vi "MSScript_Format_Start.vi"(9 "ValueArray":string[](array[string]), 10 "TagArray":string[](array[string]), 11 "MSScript in":refnum<class "MSScript.lvclass">) -> (0 "ValueErrorArray":bool[](array[boolean]), 1 "TagErrorArray":bool[](array[boolean]), 2 "ParamErrorArray":bool[](array[boolean]), 3 "Data":variant, 4 "#ofParamError":bool)   [LabVIEW 2018, in "MSScript.lvclass"]
uses:
  MSScript.lvclass
  Ctl/MSEditorParam RFStart.ctl
  MSScript.lvclass/MSScript.ctl
  MSScript_Transform_Extended.vi
  MSScript_Transform_UInt.vi
panel:
  in  "ParamValueType":T1={"freq"=0.001, "amp"=0.01, "wfmType"=0} {"amp" format="%#.3f"; "freq" format="%#.2f"}
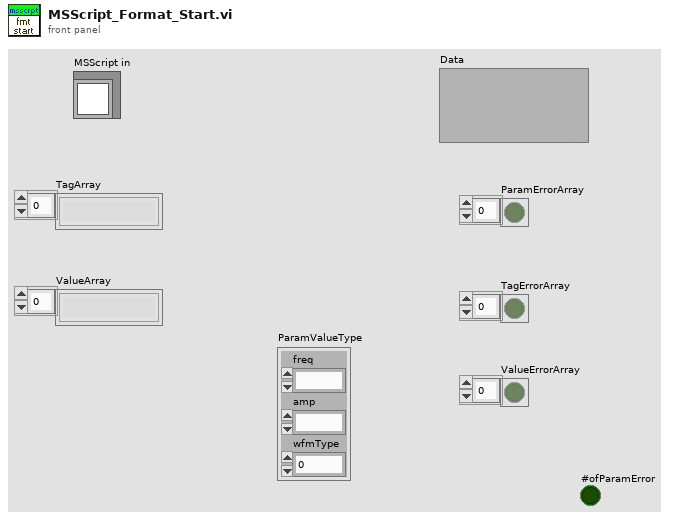
[diagram p1: front panel]
types:
  T1 = typedef "MSEditorParam RFStart.ctl" = cluster{"freq":ext, "amp":ext, "wfmType":u32}
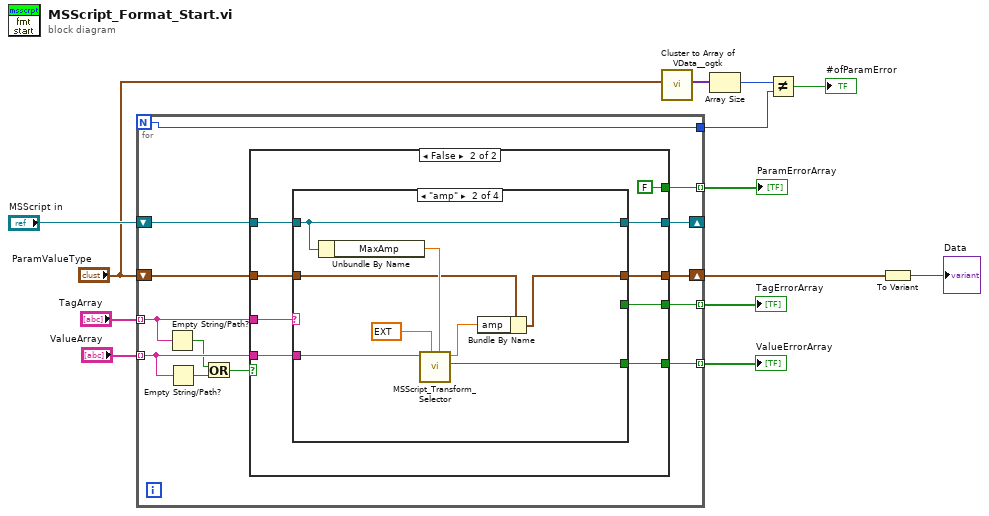
[diagram p0: block diagram]
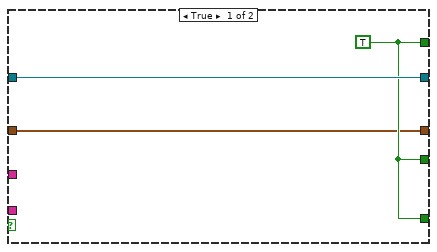
[diagram p2: hidden frame]
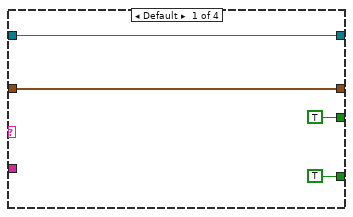
[diagram p3: hidden frame]
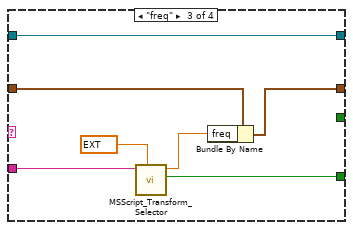
[diagram p4: hidden frame]
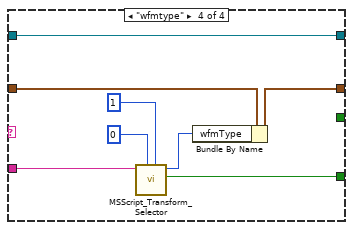
[diagram p5: hidden frame]
diagram:
  n1 = for {
    N -> [w14]
    tunnel: "TagArray" -> [w22] mode=indexing
    tunnel: "ValueArray" -> [w21] mode=indexing
    tunnel: [w26] -> w11 mode=indexing
    tunnel: [w24] -> w10 mode=indexing
    tunnel: [w17] -> w9 mode=indexing
    shift-right: [w15] -> w7
    shift-left: "ParamValueType" -> [w16]
    shift-right: [w23] -> _
    shift-left: "MSScript in" -> [w25]
    tunnel: [w14] -> w2
    n2 = Empty String/Path?(string/path=w22) -> (empty?=w19:bool)
    n3 = Empty String/Path?(string/path=w21) -> (empty?=w20:bool)
    n4 = Or(x=w19, y=w20) -> (x .or. y?=w18:bool)
    n5 = case shown="False" w18 {
      tunnel: [w28 w38] -> w26
      tunnel: w25 -> [w29 w37]
      tunnel: [w28 w36] -> w24
      tunnel: [w29 w35] -> w23
      tunnel: w22 -> [_ w34]
      tunnel: w21 -> [_ w33]
      tunnel: [w28 FALSE] -> w17
      tunnel: w16 -> [w27 w31]
      tunnel: [w27 w30] -> w15
      frame True {
        w28 = TRUE
      }
      frame False {
        n6 = case shown="\"amp\"" w34 {
          tunnel: [TRUE _ _ _] -> w38
          tunnel: w37 -> [w40 w46 w54 w63]
          tunnel: w33 -> [_ w47 w55 w64]
          tunnel: [TRUE ("Value Error?") w50 w57 w65] -> w36
          tunnel: [w40 w46 w54 w63] -> w35
          tunnel: w31 -> [w39 w44 w53 w62]
          tunnel: [w39 w43 w52 w61] -> w30
          frame Default {
          }
          frame "amp" {
            n7 = Unbundle By Name(w46) -> ("MaxAmp"=w49:ext)
            n8 = call-poly "MSScript_Transform_Selector.vi"("upper limit (Inf)"=w49, "lower limit (-Inf)"=ext 0.01 ("lower limit"), "Check_Str"=w47) -> ("Value Error?"=w50:bool, "Value Output"=w45:ext)  [unwired: 6 in, 1 out]
            n9 = Bundle By Name(cluster=w44, "amp"=w45) -> (w43:T1)
          }
          frame "freq" {
            n10 = call-poly "MSScript_Transform_Selector.vi"("lower limit (-Inf)"=ext 0.00099999999999999999996 ("lower limit"), "Check_Str"=w55) -> ("Value Error?"=w57:bool, "Value Output"=w51:ext)  [unwired: 7 in, 1 out]
            n11 = Bundle By Name(cluster=w53, "freq"=w51) -> (w52:T1)
          }
          frame "wfmtype" {
            n12 = call-poly "MSScript_Transform_Selector.vi"("upper limit"=u64 1, "lower limit"=u64 0, "string in"=w64) -> ("Value Error?"=w65:bool, "Value Output"=w60:u64)  [unwired: 6 in, 1 out]
            n13 = Bundle By Name(cluster=w62, "wfmType"=w60) -> (w61:T1)
          }
        }
      }
    }
  }
  "TagErrorArray" <- w11
  "ValueErrorArray" <- w10
  "ParamErrorArray" <- w9
  n14 = call <userlib>:"Cluster to Array of VData__ogtk.vi"("Cluster"="ParamValueType") -> ("Array of VData"=w6:variant[])  [unwired: 9 in, 1 out]
  n15 = Array Size(array=w6) -> (size(s)=w5:i32)
  n16 = Not Equal?(x=w5, y=w2) -> (x != y?=→"#ofParamError":bool)
  n17 = To Variant(anything=w7) -> (Variant=→"Data":variant)
